vi "analysis only.vi"() -> ()   [LabVIEW 2014]
panel:
  in  "change settings dir":bool
  in  "exit":bool
  in  "analyze data":bool
  # "animal version June 2010"
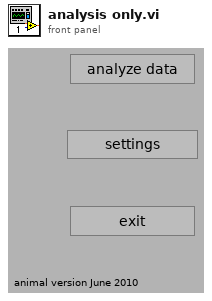
[diagram p1: front panel]
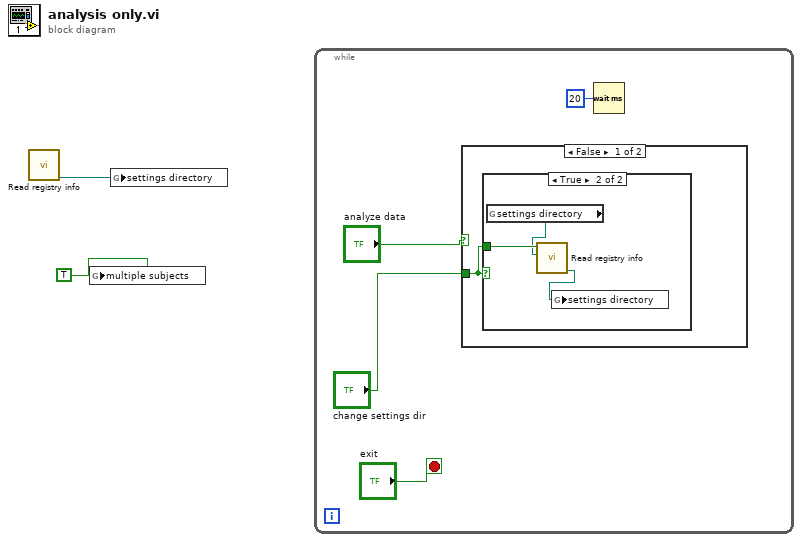
[diagram p0: block diagram]
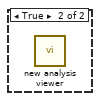
[diagram p3: hidden frame]
diagram:
  n1 = call "Read registry info.vi"() -> ("settings directory"=w2:path)  [unwired: 11 in]
  n2 = global write "acquisition globals" "multiple subjects"(TRUE ("multiple subjects")) -> ()
  n3 = global write "global settings" "settings directory"(w2) -> ()
  n4 = while {
    stop <- "exit" stop-if-true
    n5 = case shown="False" "analyze data" {
      tunnel: "change settings dir" -> [w7 _]
      frame False {
        n6 = case shown="True" w7 {
          tunnel: w7 -> [_ w10]
          frame False {
          }
          frame True {
            n7 = global read "global settings" "settings directory"() -> (w9:path)
            n8 = call "Read registry info.vi"("settings directory in"=w9, "change directory"=w10) -> ("settings directory"=w8:path)  [unwired: 9 in]
            n9 = global write "global settings" "settings directory"(w8) -> ()
          }
        }
      }
      frame True {
        n10 = call "new analysis viewer.vi"() -> ()  [unwired: 8 in]
      }
    }
    n11 = Wait (ms)(milliseconds to wait=u32 20) -> ()  [unwired: 1 out]
  }
